vi "选择产品.vi"() -> ()   [LabVIEW 2020]
panel:
  in  "不知道":T1(xcontrol)
  # "请选择产品"
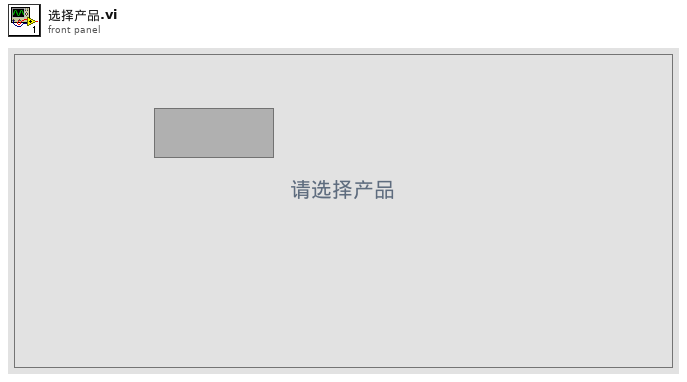
[diagram p1: front panel]
types:
  T1 = enum16{"Idle", "Runing", "Pass", "Faild", "Skip"}
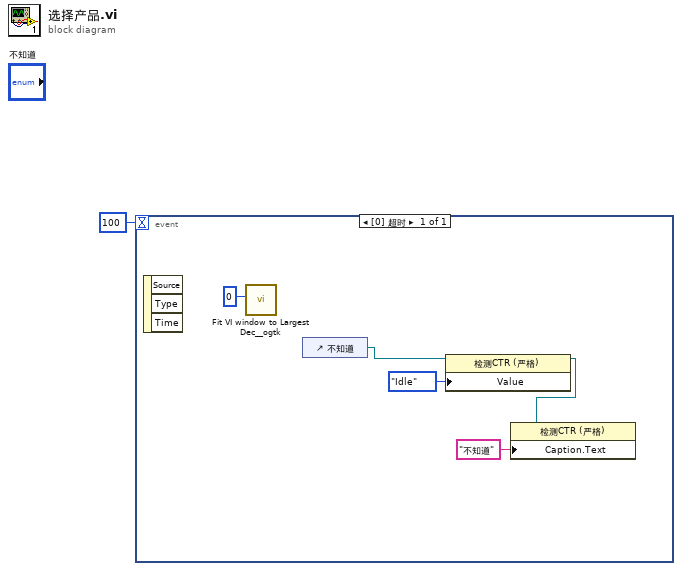
[diagram p0: block diagram]
diagram:
  n1 = event shown="[0] 超时" {
    selector: _ -> [_]
    dyn-events: _ -> [_]
    timeout: 100 -> [_]
    event Timeout {
      n2 = event-data() -> ()  [unwired: 1 in, 3 out]
      n3 = call <userlib>:"Fit VI window to Largest Dec__ogtk.vi"("border spacing (2 px)"=0) -> ()  [unwired: 5 in, 2 out]
      n4 = control-ref of="不知道"() -> (w4:refnum<vi>)
      n5 = property class="检测CTR (严格)"(reference=w4, "Value"=T1."Idle" ("值")) -> (reference out=w3:refnum<vi>)  [unwired: 1 in, 1 out]
      n6 = property class="检测CTR (严格)"(reference=w3, "Caption.Text"="不知道" ("标签.文本")) -> ()  [unwired: 1 in, 2 out]
    }
  }
